vi "ReadingParameterAddress.vi"(8 "error in (no error)":errorcluster, 10 "Адрес параметра":u16 format="%04x", 11 "StepMotor in":refnum<class "StepMotor.lvclass">) -> (0 "error out":errorcluster, 3 "StepMotor out":refnum<class "StepMotor.lvclass">)   [LabVIEW 2010, in "StepMotor.lvclass"]
doc: "Чтение параметра по адресу из СПШ."
uses:
  StepMotor.lvclass
  StepMotor.lvclass/StepMotor.ctl
panel:
  in  "Адреса параметров":u16(ring) items=["0000", "0002", "0004", "0005", "0010", "0048", "0053", "0060", "0814", "0815", "0821", "0822", "0006", "0007", "0050", "0008", "0009", "000A", "000E", "0011", "0014", "000F", "0031", "0032", "0033", "0034", "0039", "0040", "0063", "0A16", "0A17", "0A18", "0A19", "0A1A", "0A1B", "0A1C", "081F", "0820", "000B", "000C", "000D", "0012", "0041", "0A12", "0A13", "0A14", "0A15", "081C", "0013", "001F", "0020", "0021", "0022", "0023", "0024", "0025", "0026", "0027", "0028", "0029", "002A", "002B", "002C", "0600", "0601", "0818", "0819", "081A", "0200", "0202", "0204", "0400", "040A", "0405", "040D", "0402", "0408", "0409", "0419", "040B", "040C", "0418", "040E", "0417", "0410", "040F", "0411", "0412", "0413", "0414", "0415", "0416", "0420", "0421", "0422", "0423", "0424", "0425", "0426", "0427", "0428", "0429", "042A", "042B", "042C", "0015", "0016", "001E", "0046", "0047", "0802", "0804", "0062", "0816", "0817", "0823", "0824", "0825", "0826", "0500", "0504", "0502", "0505", "0506", "0017", "0018", "001A", "001B", "001C", "001D", "0030", "0035", "0036", "0037", "0038", "0042", "0045", "0057", "0058", "0059", "0061", "0800", "0801", "081D", "081E", "0043", "0044", "0051", "0052", "0054", "0056", "081B", "0700", "0701", "0702", "0703", "0704", "0705", "0706", "0707", "0708", "0709", "070A", "070B", "070C", "070D", "070E", "070F", "0710", "0711", "0712", "0713", "0714", "0715", "0716", "0717", "0718", "0805", "0806", "0807", "0808", "0809", "080A", "080B", "080C", "080D", "080E", "080F", "0810", "0811", "0812", "070F", "0A01", "0A02", "0A03", "0A04", "0A05", "0A06", "0A07", "0A08", "0A09", "0A0A", "0A0B", "0A0C", "0A0D", "0A0E", "0A0F", "0A10", "0A11", "0A1D", "0A1E", ""]
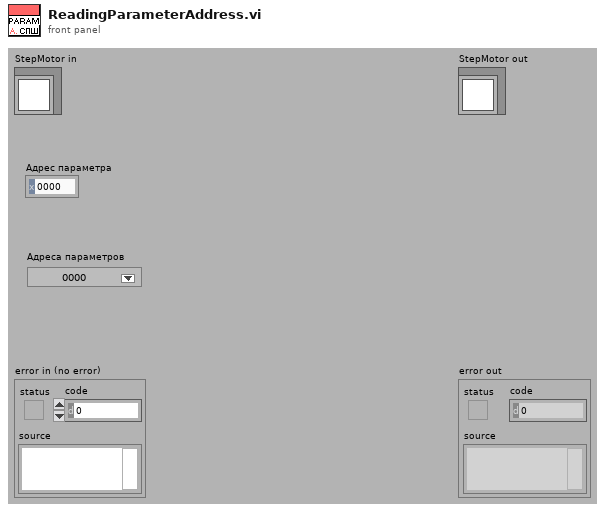
[diagram p1: front panel]
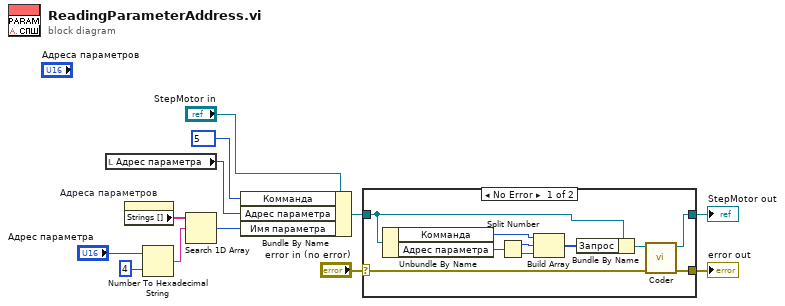
[diagram p0: block diagram]
diagram:
  n1 = local read "Адрес параметра"() -> (w2:u16)
  n2 = property on="Адреса параметров" class="Ring (strict)"() -> ("Strings []"=w6:string[])  [unwired: 2 in, 2 out]
  n3 = Number To Hexadecimal String(1:i16 4 ("width (-)"), 2:"Адрес параметра") -> (0:w5:string)
  n4 = Search 1D Array(1D array=w6, element=w5) -> (index of element=w4:i32)  [unwired: 1 in]
  n5 = Bundle By Name(cluster="StepMotor in", "Комманда"=u8 5 ("Numeric"), "Адрес параметра"=w2, "Имя параметра"=w4) -> (w11:refnum<class "StepMotor.lvclass">)
  n6 = case shown="No Error" "error in (no error)" {
    selector: "error in (no error)" -> [w16 w24]
    tunnel: [w17 w24] -> w8
    tunnel: [w18 w23] -> w9
    tunnel: w11 -> [w20 w23]
    frame No Error {
      n7 = Unbundle By Name(w20) -> ("Комманда"=w13:u8, "Адрес параметра"=w22:u16)
      n8 = Split Number(x=w22) -> (hi(x)=w15:u8, lo(x)=w14:u8)
      n9 = Build Array(w13, w15, w14) -> (w21:u8[])
      n10 = Bundle By Name(cluster=w20, "Запрос"=w21) -> (w19:refnum<class "StepMotor.lvclass">)
      n11 = call "Coder.vi"("error in (no error)"=w16, "StepMotor in"=w19) -> ("error out"=w17:errorcluster, "StepMotor out"=w18:refnum<class "StepMotor.lvclass">)  [unwired: 8 in]
    }
    frame Error {
    }
  }
  "error out" <- w8
  "StepMotor out" <- w9
